vi "Apply Configuration.vi"(8 "error in":errorcluster, 11 "Fgen Base in":refnum<class "FGEN Base.lvclass">) -> (0 "error out":errorcluster, 3 "Fgen Base out":refnum<class "FGEN Base.lvclass">)   [LabVIEW 2023, in "FGEN.lvlib" / "FGEN Base.lvlib" / "FGEN Base.lvclass"]
uses:
  FGEN Base.lvclass
  FGEN Base.lvclass/FGEN Base.ctl
  Interfaces/IConfigure/IConfigure.lvclass
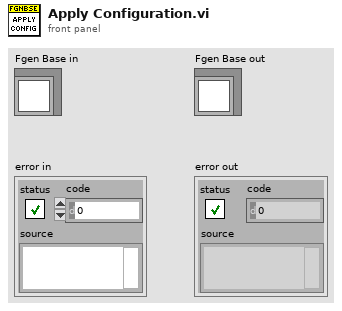
[diagram p1: front panel]
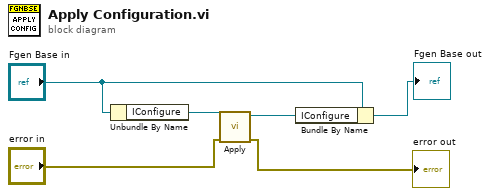
[diagram p0: block diagram]
diagram:
  n1 = Unbundle By Name("Fgen Base in") -> ("IConfigure"=w6:refnum<class "IConfigure.lvclass">)
  n2 = call-dynamic "Apply.vi"("Error In"="error in", "IConfigure in"=w6) -> ("Error Out"=→"error out":errorcluster, "IConfigure out"=w5:refnum<class "IConfigure.lvclass">)  [unwired: 8 in]
  n3 = Bundle By Name(cluster="Fgen Base in", "IConfigure"=w5) -> (→"Fgen Base out":refnum<class "FGEN Base.lvclass">)
